vi "InitScrollbarAndListBox.vi"(5 "control refs":T1, 7 "configuration":T2, 8 "error in (no error)":errorcluster, 9 "channel names":string[](array[string]), 10 "group names":string[](array[string]), 11 "tdms in":refnum<k34>) -> (0 "error out":errorcluster, 1 "channel out":string[](array[string]), 2 "group out":string[](array[string]), 3 "tdms out":refnum<k34>)   [LabVIEW 2020]
uses:
  <vilib>/Utility/tdmsutil.llb/fileViewerConfigData.ctl
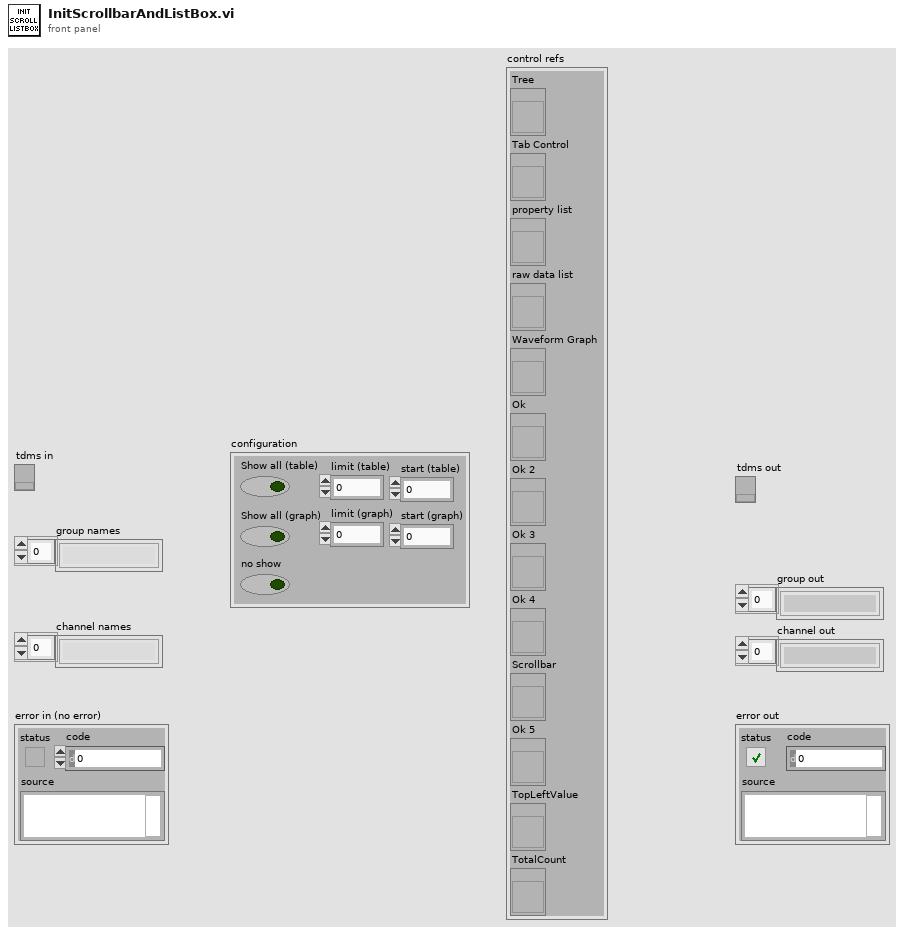
[diagram p1: front panel]
types:
  T1 = cluster{"Tree":refnum<vi>, "Tab Control":refnum<vi>, "property list":refnum<vi>, "raw data list":refnum<vi>, "Waveform Graph":refnum<vi>, "Ok":refnum<vi>, "Ok 2":refnum<vi>, "Ok 3":refnum<vi>, "Ok 4":refnum<vi>, "Scrollbar":refnum<vi>, "Ok 5":refnum<vi>, "TopLeftValue":refnum<vi>, "TotalCount":refnum<vi>}
  T2 = typedef "fileViewerConfigData.ctl" = cluster{"Show all (table)":bool, "Show all (graph)":bool, "limit (table)":u64, "limit (graph)":u64, "no show":bool, "start (table)":u64, "start (graph)":u64}
  T3 = typedef "LVRowAndColumnUnsignedTypeDef.ctl" = cluster{"Row":u32, "Column":u32}
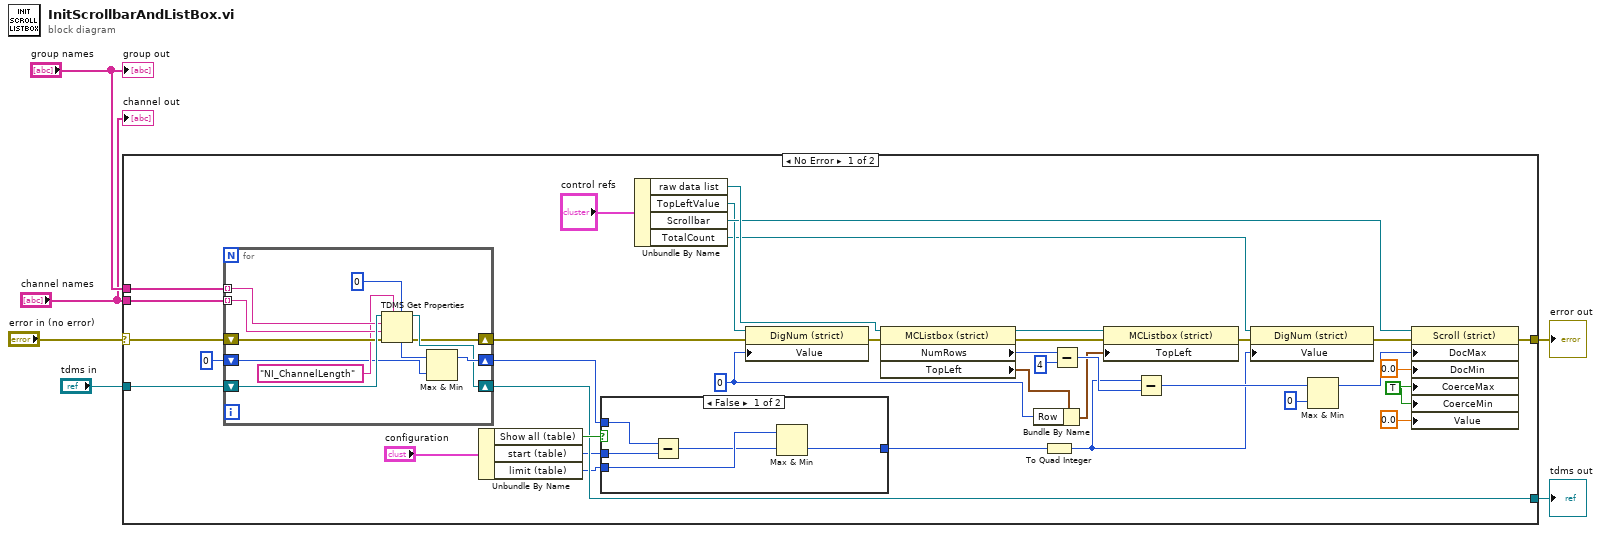
[diagram p0: block diagram]
diagram:
  n1 = case shown="No Error" "error in (no error)" {
    selector: "error in (no error)" -> [w12 w61]
    tunnel: [w41 w62] -> w6
    tunnel: "tdms in" -> [w37 w62]
    tunnel: "group names" -> [w36 _]
    tunnel: "channel names" -> [w34 _]
    tunnel: [w13 w61] -> w2
    frame No Error {
      w21 = u64 0 ("LastLeftTopRow")
      w33 = TRUE ("Coerce Maximum Value")
      n2 = for {
        tunnel: w36 -> [w53] mode=indexing
        tunnel: w34 -> [w52] mode=indexing
        shift-right: [w46] -> w40
        shift-left: u64 0 -> [w47]
        shift-right: [w44] -> w16
        shift-left: w12 -> [w51]
        shift-right: [w45] -> w41
        shift-left: w37 -> [w54]
        n3 = TDMS Get Properties(5:u64 0, 7:"NI_ChannelLength" ("property name"), 8:w51, 9:w52, 10:w53, 11:w54) -> (0:w44:errorcluster, 3:w45:refnum<k34>, 4:w48:u64)  [unwired: 3 out]
        n4 = Max & Min(x=w48, y=w47) -> (max(x,y)=w46:u64)  [unwired: 1 out]
      }
      n5 = Unbundle By Name("configuration") -> ("Show all (table)"=w43:bool, "start (table)"=w38:u64, "limit (table)"=w39:u64)
      n6 = case shown="False" w43 {
        tunnel: w40 -> [w58 w60]
        tunnel: w39 -> [w59 _]
        tunnel: w38 -> [w57 _]
        tunnel: [w55 w60] -> w18
        frame False {
          n7 = Subtract(x=w58, y=w57) -> (x-y=w56:u64)
          n8 = Max & Min(x=w59, y=w56) -> (min(x,y)=w55:u64)  [unwired: 1 out]
        }
        frame True {
        }
      }
      n9 = Unbundle By Name("control refs") -> ("raw data list"=w24:refnum<vi>, "TopLeftValue"=w22:refnum<vi>, "Scrollbar"=w23:refnum<vi>, "TotalCount"=w10:refnum<vi>)
      n10 = property class="DigNum (strict)"(reference=w22, error in=w16, "Value"=w21) -> (error out=w15:errorcluster)  [unwired: 1 out]
      n11 = property on="Property Node" class="MCListbox (strict)"(reference=w24, error in=w15) -> (reference out=w17:refnum<vi>, error out=w14:errorcluster, "NumRows"=w27:u32, "TopLeft"=w20:T3)
      n12 = Bundle By Name(cluster=w20, "Row"=w21) -> (w19:T3)
      n13 = To Quad Integer(1:w18) -> (0:w7:i64)
      n14 = Subtract(x=w27, y=u32 4) -> (x-y=w25:u32)
      n15 = property on="Property Node" class="MCListbox (strict)"(reference=w17, error in=w14, "TopLeft"=w19) -> (error out=w9:errorcluster)  [unwired: 1 out]
      n16 = Subtract(x=w7, y=w25) -> (x-y=w30:i64)
      n17 = property class="DigNum (strict)"(reference=w10, error in=w9, "Value"=w7) -> (error out=w8:errorcluster)  [unwired: 1 out]
      n18 = Max & Min(x=w30, y=i64 0) -> (max(x,y)=w28:i64)  [unwired: 1 out]
      n19 = property on="Property Node" class="Scroll (strict)"(reference=w23, error in=w8, "DocMax"=w28, "DocMin"=0.0 ("Doc Min"), "CoerceMax"=w33, "CoerceMin"=w33, "Value"=0.0 ("Scrollbar")) -> (error out=w13:errorcluster)  [unwired: 1 out]
    }
    frame Error {
    }
  }
  "error out" <- w2
  "tdms out" <- w6
  "group out" <- "group names"
  "channel out" <- "channel names"
